vi "Send Metronome Shutdown.vi"(8 "error in (no error)":errorcluster, 11 "Actor in":refnum<class "Actor.lvclass">) -> (0 "error out":errorcluster)   [LabVIEW 2020, in "Actor.lvclass"]
uses:
  Actor.lvclass
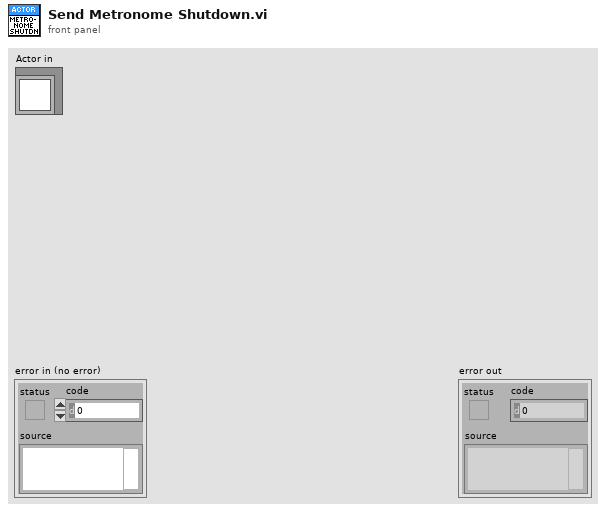
[diagram p1: front panel]
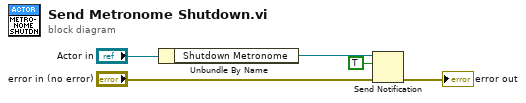
[diagram p0: block diagram]
diagram:
  n1 = Unbundle By Name("Actor in") -> ("Shutdown Metronome"=w2:refnum<notifier>)
  n2 = Send Notification(notification=TRUE, notifier=w2, error in (no error)="error in (no error)") -> (error out=→"error out":errorcluster)  [unwired: 1 out]
